vi "take the ball (SubVI).vi"(7 "Numeric":i8, 8 "error in (no error)":errorcluster, 11 "KNR in":T1) -> (0 "error out":errorcluster, 3 "KNR out":T1)   [LabVIEW 2013]
uses:
  <userlib>/KNR OS 3.0 LabVIEW Toolkit/Type Definition/KNR3 Reference.ctl
  <userlib>/_FPGA Interface Advanced Tools/FPGA Interface Base/FPGA Interface Base.lvclass
  <userlib>/KNR OS 3.0 LabVIEW Toolkit/Type Definition/Resource.ctl
  <userlib>/KNR OS 3.0 LabVIEW Toolkit/LEGO-specific Sensors/Complete Digital Sensors/Read Lego Ultrasonar Sensor.vi
panel:
  in  "STOP 2":bool
  in  "STOP":bool
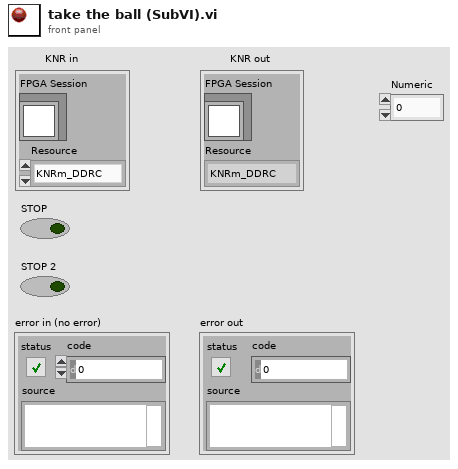
[diagram p1: front panel]
types:
  T1 = typedef "KNR3 Reference.ctl" = cluster{"FPGA Session":refnum<class "FPGA Interface Base.lvclass">, "Resource":T2}
  T2 = typedef "Resource.ctl" = enum16{"KNRm_DDRC", "KNRm_DDDD", "KNRm_DDDR", "KNRm_DDDC", "KNR"}
  T3 = typedef "Lego Port.ctl" = enum8{"L1", "LS1", "LS3", "LS4", "LS2"}
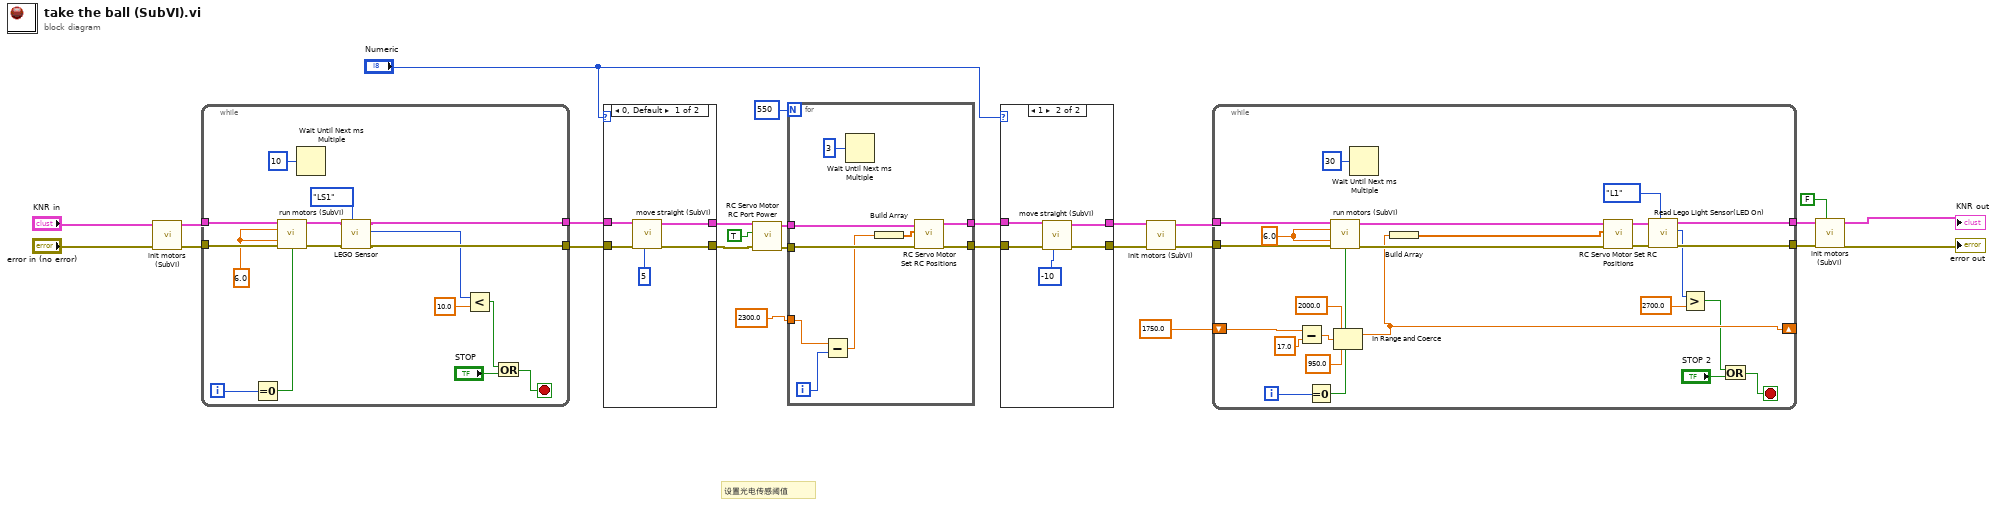
[diagram p0: block diagram]
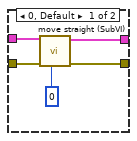
[diagram p2: hidden frame]
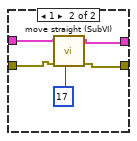
[diagram p3: hidden frame]
diagram:
  # "设置光电传感阈值"
  n1 = call "init motors (SubVI).vi"("error in (no error)"="error in (no error)", "KNR in"="KNR in") -> ("error out"=w4:errorcluster, "KNR out"=w3:T1)  [unwired: 6 in, 2 out]
  n2 = while {
    tunnel: w3 -> [w42]
    tunnel: w4 -> [w41]
    tunnel: [w29] -> w6
    tunnel: [w28] -> w5
    i -> [w37]
    stop <- w40 stop-if-true
    w34 = 6.0 ("speed_1")
    n3 = Equal To 0?(x=w37) -> (x = 0?=w36:bool)
    n4 = call "run motors (SubVI).vi"("KNR in"=w42, "speed_1"=w34, "speed_2"=w34, "error in (no error)"=w41, "reinitialize? (F)"=w36) -> ("KNR out 2"=w31:T1, "error out"=w30:errorcluster)  [unwired: 7 in, 2 out]
    n5 = Wait Until Next ms Multiple(millisecond multiple=u32 10) -> ()  [unwired: 1 out]
    n6 = call-poly <userlib>:"LEGO Sensor.vi"("Port (LS1)"=Lego_Port."LS1", "error in (no error)"=w30, "KNR in"=w31) -> ("error out"=w29:errorcluster, "distance(cm)"=w27:u8, "KNR out"=w28:T1)  [unwired: 6 in]
    n7 = Less?(x=w27, y=10.0) -> (x < y?=w39:bool)
    n8 = Or(x=w39, y="STOP") -> (x .or. y?=w40:bool)
  }
  n9 = case shown="0, Default" "Numeric" {
    tunnel: w5 -> [w46 w49]
    tunnel: w6 -> [w47 w48]
    tunnel: [w44 w51] -> w8
    tunnel: [w43 w50] -> w9
    frame 0, Default {
      n10 = call "move straight (SubVI).vi"("DST"=5, "error in (no error)"=w47, "KNR in"=w46) -> ("error out"=w43:errorcluster, "KNR out"=w44:T1)  [unwired: 7 in]
    }
    frame 1 {
      n11 = call "move straight (SubVI).vi"("DST"=17, "error in (no error)"=w48, "KNR in"=w49) -> ("error out"=w50:errorcluster, "KNR out"=w51:T1)  [unwired: 7 in]
    }
  }
  n12 = call <userlib>:"RC Servo Motor RC Port Power.vi"("error in (no error)"=w9, "RC Power(F)"=TRUE, "KNR in"=w8) -> ("error out"=w11:errorcluster, "KNR out"=w10:T1)  [unwired: 7 in]
  n13 = for {
    N: 550 -> [_]
    tunnel: w10 -> [w60]
    tunnel: w11 -> [w59]
    tunnel: 2300.0 ("element") -> [w58]
    tunnel: [w54] -> w15
    tunnel: [w53] -> w14
    i -> [w57]
    n14 = Subtract(x=w58, y=w57) -> (x-y=w55:dbl)
    n15 = Wait Until Next ms Multiple(millisecond multiple=u32 3) -> ()  [unwired: 1 out]
    n16 = Build Array(w55) -> (w61:dbl[])
    n17 = call <userlib>:"RC Servo Motor Set RC Positions.vi"("error in (no error)"=w59, "RC Pulse Width (1500 uS)"=w61, "KNR in"=w60) -> ("error out"=w53:errorcluster, "KNR out"=w54:T1)  [unwired: 7 in]
  }
  n18 = case shown="1" "Numeric" {
    tunnel: w15 -> [w65 w70]
    tunnel: w14 -> [w66 w69]
    tunnel: [w63 w68] -> w17
    tunnel: [w62 w67] -> w18
    frame 0, Default {
      n19 = call "move straight (SubVI).vi"("DST"=0, "error in (no error)"=w66, "KNR in"=w65) -> ("error out"=w62:errorcluster, "KNR out"=w63:T1)  [unwired: 7 in]
    }
    frame 1 {
      n20 = call "move straight (SubVI).vi"("DST"=-10, "error in (no error)"=w69, "KNR in"=w70) -> ("error out"=w67:errorcluster, "KNR out"=w68:T1)  [unwired: 7 in]
    }
  }
  n21 = call "init motors (SubVI).vi"("error in (no error)"=w18, "KNR in"=w17) -> ("error out"=w20:errorcluster, "KNR out"=w19:T1)  [unwired: 6 in, 2 out]
  n22 = while {
    tunnel: w19 -> [w96]
    tunnel: w20 -> [w95]
    tunnel: [w88] -> w23
    tunnel: [w87] -> w22
    shift-right: [w78] -> _
    shift-left: 1750.0 ("element") -> [w81]
    i -> [w92]
    stop <- w94 stop-if-true
    w89 = 6.0 ("speed_1")
    n23 = Subtract(x=w81, y=17.0) -> (x-y=w79:dbl)
    n24 = Equal To 0?(x=w92) -> (x = 0?=w91:bool)
    n25 = call "run motors (SubVI).vi"("KNR in"=w96, "speed_1"=w89, "speed_2"=w89, "error in (no error)"=w95, "reinitialize? (F)"=w91) -> ("KNR out 2"=w83:T1, "error out"=w82:errorcluster)  [unwired: 7 in, 2 out]
    n26 = In Range and Coerce(upper limit=2000.0, x=w79, lower limit=950.0) -> (coerced(x)=w78:dbl)  [unwired: 1 out]
    n27 = Wait Until Next ms Multiple(millisecond multiple=u32 30) -> ()  [unwired: 1 out]
    n28 = Build Array(w78) -> (w86:dbl[])
    n29 = call <userlib>:"RC Servo Motor Set RC Positions.vi"("error in (no error)"=w82, "RC Pulse Width (1500 uS)"=w86, "KNR in"=w83) -> ("error out"=w84:errorcluster, "KNR out"=w85:T1)  [unwired: 7 in]
    n30 = call <userlib>:"Read Lego Light Sensor(LED On).vi"("Port (LS2)"=Lego_Port."L1", "error in (no error)"=w84, "KNR in"=w85) -> ("error out"=w87:errorcluster, "Row Value"=w72:u16, "KNR out"=w88:T1)  [unwired: 5 in, 1 out]
    n31 = Greater?(x=w72, y=2700.0) -> (0:w73:bool)
    n32 = Or(x=w73, y="STOP 2") -> (x .or. y?=w94:bool)
  }
  n33 = call "init motors (SubVI).vi"("Enable Motor(T)"=FALSE, "error in (no error)"=w22, "KNR in"=w23) -> ("error out"=→"error out":errorcluster, "KNR out"=→"KNR out":T1)  [unwired: 5 in, 2 out]
